vi "calculate tomo progress.vi"(8 "error in (no error)":errorcluster, 11 "Autofocus in":refnum<class "Autofocus.lvclass">) -> (0 "error out":errorcluster, 3 "Autofocus out":refnum<class "Autofocus.lvclass">)   [LabVIEW 2012, in "Autofocus.lvclass"]
uses:
  Autofocus.lvclass
  Autofocus.lvclass/Autofocus.ctl
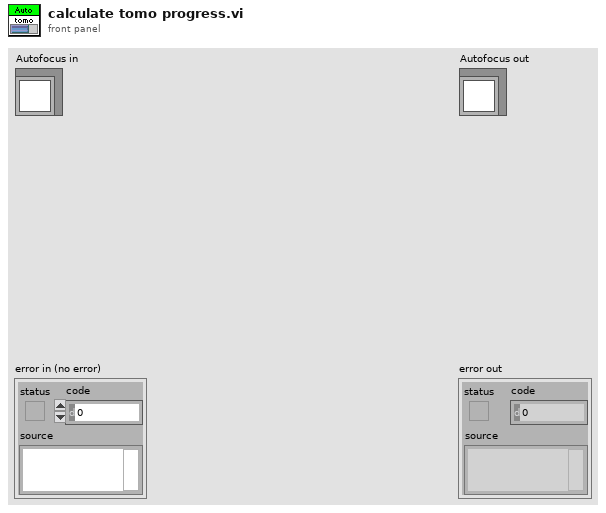
[diagram p1: front panel]
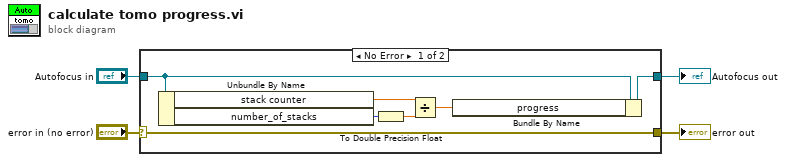
[diagram p0: block diagram]
diagram:
  n1 = case shown="No Error" "error in (no error)" {
    selector: "error in (no error)" -> [w11 w13]
    tunnel: [w11 w13] -> w3
    tunnel: [w6 w12] -> w1
    tunnel: "Autofocus in" -> [w7 w12]
    frame No Error {
      n2 = Unbundle By Name(w7) -> ("stack counter"=w10:dbl, "number_of_stacks"=w9:u16)
      n3 = To Double Precision Float(number=w9) -> (double precision float=w8:dbl)
      n4 = Divide(x=w10, y=w8) -> (x/y=w5:dbl)
      n5 = Bundle By Name(cluster=w7, "progress"=w5) -> (w6:refnum<class "Autofocus.lvclass">)
    }
    frame Error {
    }
  }
  "error out" <- w3
  "Autofocus out" <- w1
